vi "Convert(SubVI).vi"(1 "Left Thumbstick.X Axis":i32) -> (0 "Numeric":u8)   [LabVIEW 2019]
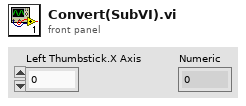
[diagram p1: front panel]
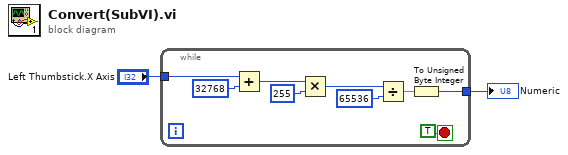
[diagram p0: block diagram]
diagram:
  n1 = while {
    tunnel: [w11] -> w2
    tunnel: "Left Thumbstick.X Axis" -> [w5]
    stop <- TRUE stop-if-true
    n2 = Add(x=w5, y=32768 ("Left Thumbstick.X Axis")) -> (x+y=w6:i32)
    n3 = Multiply(x=w6, y=255 ("Left Thumbstick.X Axis")) -> (x*y=w8:i32)
    n4 = Divide(x=w8, y=65536 ("Left Thumbstick.X Axis")) -> (x/y=w10:dbl)
    n5 = To Unsigned Byte Integer(number=w10) -> (unsigned 8bit integer=w11:u8)
  }
  "Numeric" <- w2
